vi "Write OSF Token.vi"(8 "error in (no error)":errorcluster, 10 "Token":string, 11 "Log Record in":refnum<class "Log Record.lvclass">) -> (0 "error out":errorcluster, 3 "Log Record out":refnum<class "Log Record.lvclass">)   [LabVIEW 2020, in "Log Record.lvclass"]
uses:
  Log Record.lvclass
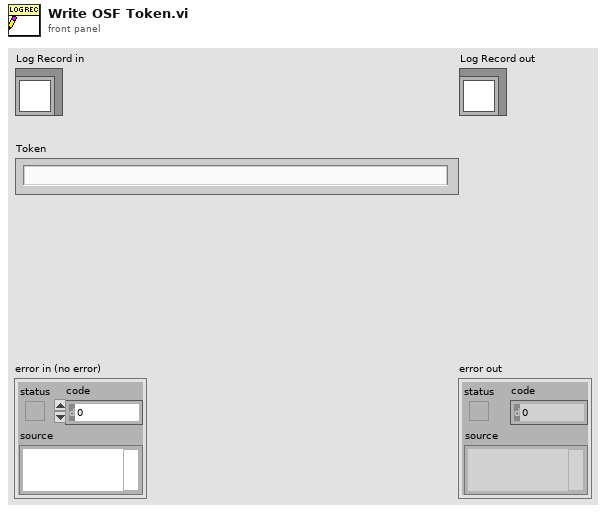
[diagram p1: front panel]
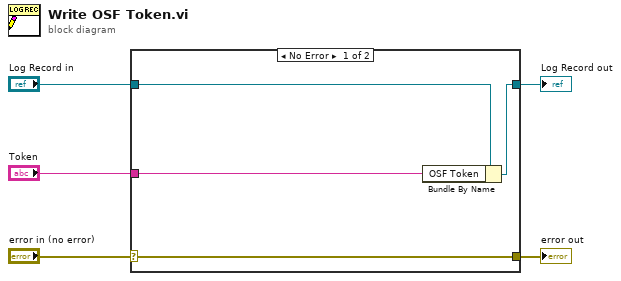
[diagram p0: block diagram]
diagram:
  n1 = case shown="No Error" "error in (no error)" {
    selector: "error in (no error)" -> [w9 w10]
    tunnel: [w9 w10] -> w4
    tunnel: [w7 w11] -> w2
    tunnel: "Log Record in" -> [w8 w11]
    tunnel: "Token" -> [w6 _]
    frame No Error {
      n2 = Bundle By Name(cluster=w8, "OSF Token"=w6) -> (w7:refnum<class "Log Record.lvclass">)
    }
    frame Error {
    }
  }
  "error out" <- w4
  "Log Record out" <- w2
